vi "Temp1,2,3,4,5y6.vi"() -> ()   [LabVIEW 2023]
uses:
  <vilib>/MakerHub/LINX/LMH-LINX.lvlib
  <vilib>/MakerHub/LINX/Public/Peripherals/Analog/Analog Read 1 Chan.vi
  <vilib>/MakerHub/LINX/Public/Peripherals/Digital/Digital Write 1 Chan.vi
  <vilib>/MakerHub/LINX/Public/Utilities/Open Serial.vi
panel:
  out "on/off":bool
  in  "Serial Port":refnum<visa-resource-name>="N/A"
  in  "stop":bool
  out "Numeric":dbl
  out "Thermometer":dbl(slide) scale=0.0..100.0
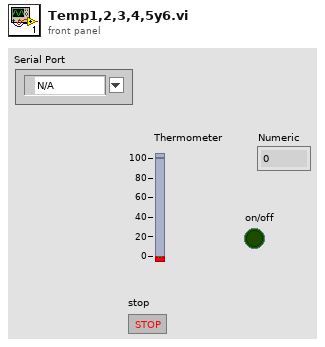
[diagram p1: front panel]
types:
  T1 = typedef "LMH-LINX.lvlib/LINX Ref.ctl" = cluster{"IO":T2, "Interface":T3, "LINX Device Config":T4}
  T2 = typedef "LMH-LINX.lvlib/Platform.ctl" = enum16{"Remote", "Local"}
  T3 = typedef "LMH-LINX.lvlib/Interface.ctl" = enum16{"Serial", "TCP"}
  T4 = typedef "LMH-LINX.lvlib/Device.lvlib/LINX Device Config.ctl" = cluster{"Interface":T3, "COM Port":refnum<visa-resource-name>, "TCP Configuration":T5, "Device Family":u8, "Device ID":u8, "Device Name":string, "TCP Ref":refnum<k5>, "Channels":T6}
  T5 = typedef "LMH-LINX.lvlib/Device.lvlib/TCP Config.ctl" = cluster{"IP Address":string, "Port":u16}
  T6 = typedef "LMH-LINX.lvlib/Channels.ctl" = cluster{"DI":u8[], "DO":u8[], "AI":u8[], "AO":u8[], "PWM":u8[], "QE":u8[], "UART":u8[], "I2C 2":u8[], "SPI":u8[], "CAN":u8[], "Servo":u8[], "AI Ref (V)":dbl, "AI Resolution (Bits)":u8, "AO Ref (V)":dbl, "AO Resolution (Bits)":u8}
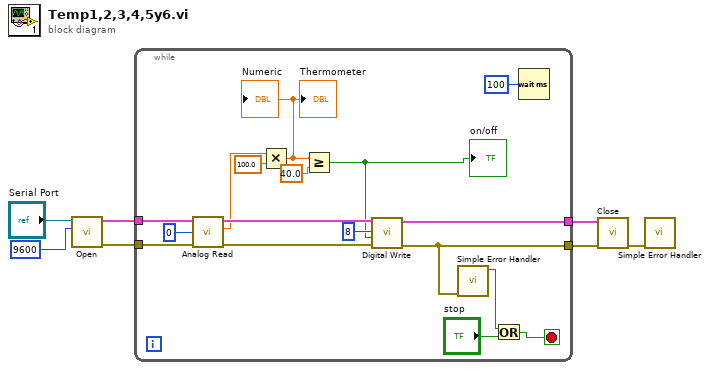
[diagram p0: block diagram]
diagram:
  n1 = call-poly <vilib>:"Open.vi"("Baud Rate Override"=u32 9600, "Serial Port"="Serial Port") -> ("Error Out"=w5:errorcluster, "LINX Resource"=w6:T1)  [unwired: 7 in, 1 out]
  n2 = while {
    tunnel: [w9] -> w7
    tunnel: w6 -> [w19]
    tunnel: w5 -> [w18]
    tunnel: [w8] -> w1
    stop <- w24 stop-if-true
    n3 = call-poly <vilib>:"Analog Read.vi"("Error In"=w18, "Analog Channel"=u8 0, "LINX Resource"=w19) -> ("Error Out"=w21:errorcluster, "Voltage"=w14:dbl, "LINX Resource"=w20:T1)  [unwired: 5 in, 1 out]
    n4 = Multiply(x=w14, y=100.0 ("x")) -> (x*y=w12:dbl)
    "Thermometer" <- w12
    "Numeric" <- w12
    n5 = Greater Or Equal?(x=w12, y=40.0) -> (x >= y?=w11:bool)
    "on/off" <- w11
    n6 = call-poly <vilib>:"Digital Write.vi"("Error In"=w21, "Output Value"=w11, "DO Channel"=u8 8, "LINX Resource"=w20) -> ("Error Out"=w8:errorcluster, "LINX Resource"=w9:T1)  [unwired: 6 in]
    n7 = call <vilib>:"Simple Error Handler.vi"("error in (no error)"=w8) -> ("error?"=w10:bool)  [unwired: 4 in, 4 out]
    n8 = Or(x=w10, y="stop") -> (x .or. y?=w24:bool)
    n9 = Wait (ms)(milliseconds to wait=u32 100) -> ()  [unwired: 1 out]
  }
  n10 = call <vilib>:"Close.vi"("Error In"=w1, "LINX Resource"=w7) -> ("Error Out"=w2:errorcluster)  [unwired: 9 in]
  n11 = call <vilib>:"Simple Error Handler.vi"("error in (no error)"=w2) -> ()  [unwired: 4 in, 5 out]
